vi "MeasAction.vi"(8 "error in (no error)":errorcluster caption="entrée d'erreur (pas d'erreur)", 9 "CurvePointIndex":i32, 10 "AllPointIndex":i32, 11 "InstrClassIn":refnum<class "CoboltMLD.lvclass"> caption="DNL_LabVIEW Object in") -> (0 "error out":errorcluster caption="sortie d'erreur", 2 "MeasDatOut":dbl[](array[numeric]), 3 "InstrClassOut":refnum<class "CoboltMLD.lvclass"> caption="DNL_LabVIEW Object out")   [LabVIEW 2019, in "CoboltMLD.lvclass"]
uses:
  CoboltMLD.lvclass
  CoboltMLD.lvclass/CoboltMLD.ctl
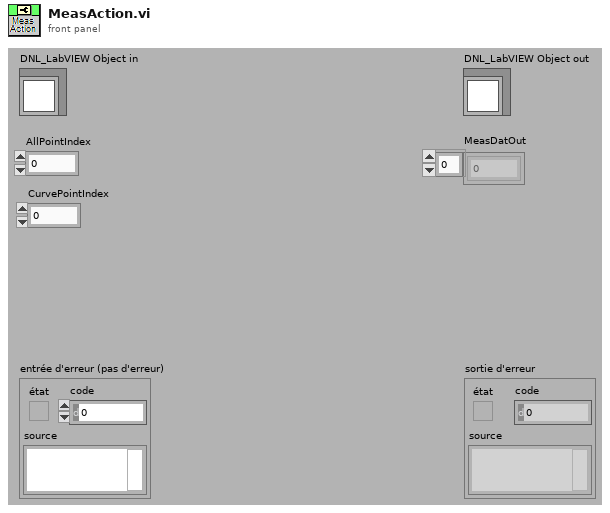
[diagram p1: front panel]
types:
  T1 = typedef "CoboltMLD.lvclass/CoboltMLD_Func.ctl" = enum16{"Power (mW)", "Current (mA)"}
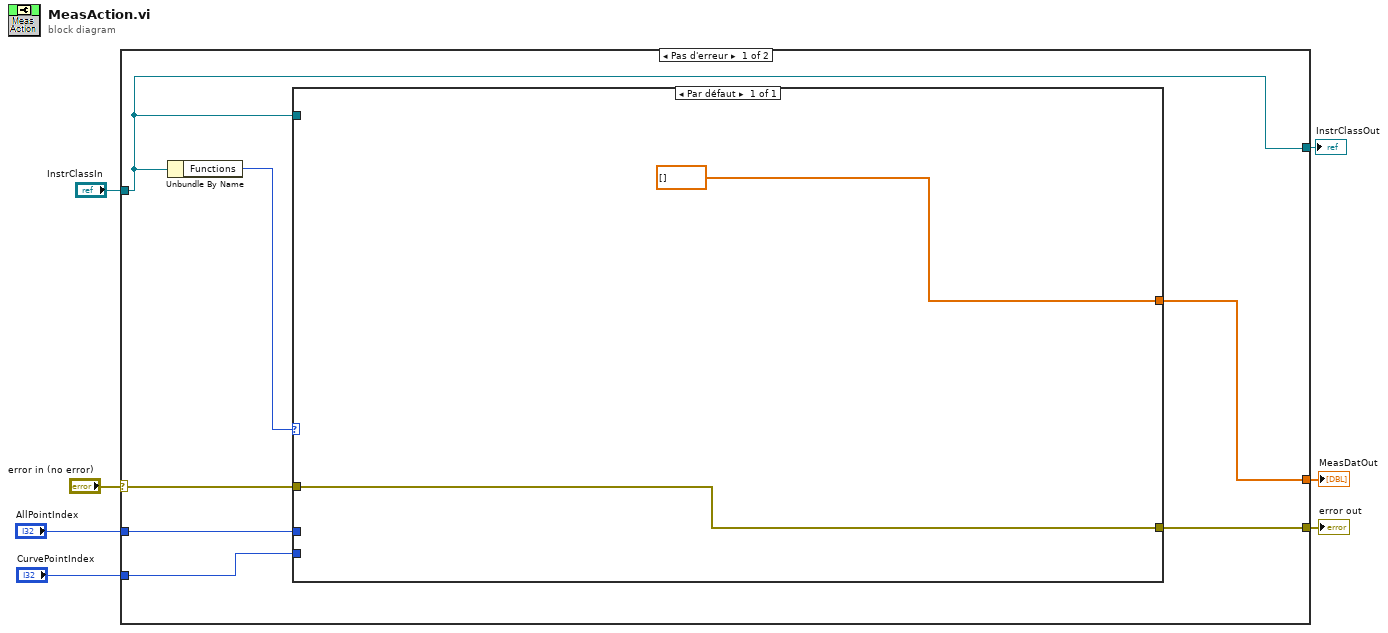
[diagram p0: block diagram]
diagram:
  n1 = case shown="Pas d'erreur" "error in (no error)" {
    selector: "error in (no error)" -> [w10 w17]
    tunnel: "InstrClassIn" -> [w8 w18]
    tunnel: [w8 w18] -> w5
    tunnel: "AllPointIndex" -> [w14 _]
    tunnel: [w13 w17] -> w3
    tunnel: [w12 _] -> w2
    tunnel: "CurvePointIndex" -> [w9 _]
    frame No Error {
      n2 = Unbundle By Name(w8) -> ("Functions"=w11:T1)
      n3 = case shown="Par défaut" w11 {
        tunnel: w14 -> [_]
        tunnel: [w15] -> w13
        tunnel: [dbl[] [] ("Outputs")] -> w12
        tunnel: w10 -> [w15]
        tunnel: w9 -> [_]
        tunnel: w8 -> [_]
        frame Par défaut {
        }
      }
    }
    frame Error {
    }
  }
  "error out" <- w3
  "InstrClassOut" <- w5
  "MeasDatOut" <- w2
